vi "lvcsm Delete Section.vi"(5 "Sub-section (\"\")":string, 6 "Config Path":path, 7 "Section":string, 8 "Error In":errorcluster caption="error in (no error)") -> (0 "error out":errorcluster)   [LabVIEW 2017, in "lvcsm File Support.lvlib"]
uses:
  lvcsm File Support.lvlib
  <vilib>/Utility/config.llb/NI_LVConfig.lvlib
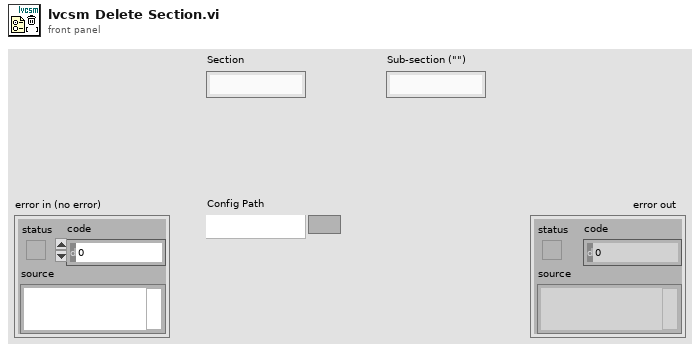
[diagram p1: front panel]
types:
  T1 = typedef "NI_LVConfig.lvlib/Config Data RefNum.ctl" = refnum<k1>
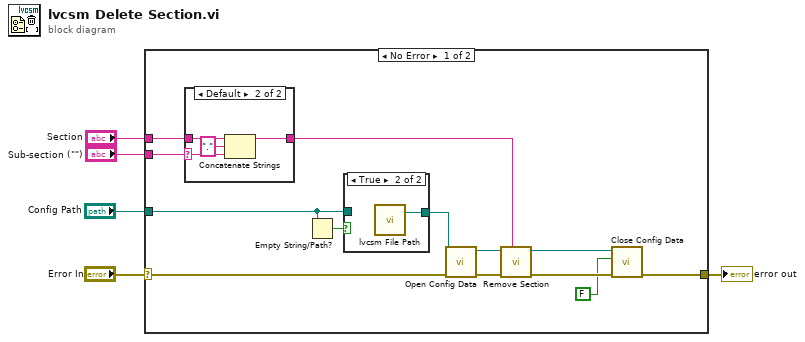
[diagram p0: block diagram]
diagram:
  n1 = case shown="No Error" "Error In" {
    selector: "Error In" -> [w7 w26]
    tunnel: "Sub-section (\"\")" -> [w18 _]
    tunnel: "Section" -> [w17 _]
    tunnel: "Config Path" -> [w15 _]
    tunnel: [w14 w26] -> w1
    frame No Error {
      n2 = case shown="Default" w18 {
        selector: w18 -> [_ w23]
        tunnel: w17 -> [w21 w25]
        tunnel: [w21 w24] -> w16
        frame "" {
        }
        frame Default {
          n3 = Concatenate Strings(w25, "." ("string"), w23) -> (w24:string)
        }
      }
      n4 = Empty String/Path?(string/path=w15) -> (empty?=w13:bool)
      n5 = case shown="True" w13 {
        tunnel: [w19 w20] -> w12
        tunnel: w15 -> [w19 _]
        frame False {
        }
        frame True {
          n6 = call "lvcsm File Path.vi"() -> ("Appended Path"=w20:path)  [unwired: 3 in]
        }
      }
      n7 = call <vilib>:"Open Config Data.vi"("error in (no error)"=w7, "configuration file path"=w12) -> ("error out"=w6:errorcluster, "refnum"=w11:T1)  [unwired: 7 in, 1 out]
      n8 = call <vilib>:"Remove Section.vi"("section"=w16, "error in (no error)"=w6, "refnum"=w11) -> ("error out"=w10:errorcluster, "refnum out"=w9:T1)  [unwired: 6 in, 1 out]
      n9 = call <vilib>:"Close Config Data.vi"("error in (no error)"=w10, "write file if changed (T)"=FALSE, "refnum"=w9) -> ("error out"=w14:errorcluster)  [unwired: 7 in, 1 out]
    }
    frame Error {
    }
  }
  "error out" <- w1
